vi "SAHarmonicDistortionToneConfigureSweepTimeAutoEnabled.vi"(8 "error in (no error)":errorcluster {"code" format="%.0x"}, 9 "State (Off)":bool, 10 "HarmonicNumber":i32=1 caption="HarmonicNumber (1)" format="%.0g", 11 "instrument handle":refnum<k15>) -> (0 "error out":errorcluster {"code" format="%.0x"}, 3 "instrument handle out":refnum<k15>)   [LabVIEW 2009, in "Keysight XSAn.lvlib"]
doc: "Sets whether the selected harmonic sweep time is set automatically or manually.\n\nSupported Models: M9290A, N8973B, N8974B, N8975B, N8976B, N9000A, N9000B, N9010A, N9010B, N9020A, N9020B, N9030A, N9030B, N9038A, N9040B, N9041B, SPN9003A, SPN9026A"
uses:
  <instrlib>/Keysight XSAn/Keysight XSAn.lvlib
  AgXSAn.dll
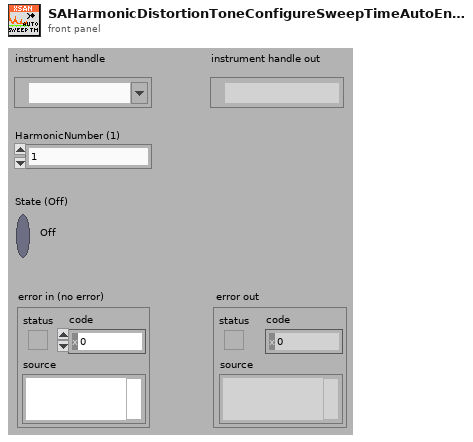
[diagram p1: front panel]
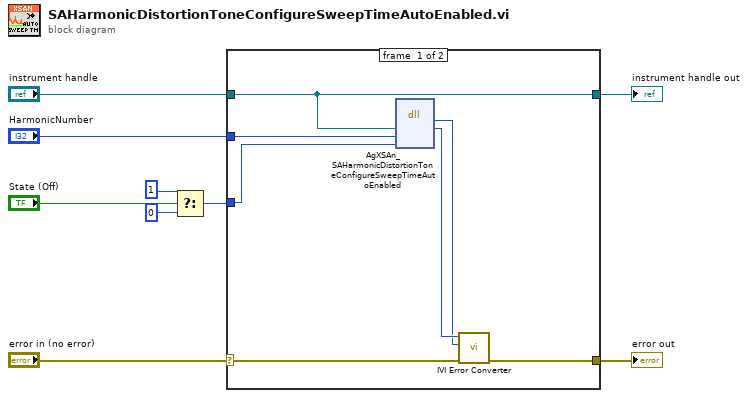
[diagram p0: block diagram]
diagram:
  n1 = Select(t=u16 1, s="State (Off)", f=u16 0) -> (s? t:f=w2:u16)
  n2 = case shown="No Error" "error in (no error)" {
    selector: "error in (no error)" -> [w14 w18]
    tunnel: [w13 w18] -> w9
    tunnel: "instrument handle" -> [w10 w17]
    tunnel: "HarmonicNumber" -> [w12 _]
    tunnel: w2 -> [w11 _]
    tunnel: [w10 w17] -> w1
    frame #0 {
      n3 = dll-call lib="AgXSAn**.dll" fn="AgXSAn_SAHarmonicDistortionToneConfigureSweepTimeAutoEnabled"("Vi"=w10, "HarmonicNumber"=w12, "State"=w11) -> (w15:i32, "Vi"=w16:u32)  [unwired: 5 in, 2 out]
      n4 = call <instrlib>:"IVI Error Converter.vi"("error in (no error)"=w14, "IVI error code (0)"=w15, "instrument handle"=w16) -> ("error out"=w13:errorcluster)  [unwired: 7 in, 1 out]
    }
    frame #1 {
    }
  }
  "error out" <- w9
  "instrument handle out" <- w1
